vi "CAN Frame Filter.vi"(10 "Filter":T3, 11 "frames in":T4[](array[typedef]) {"payload" format="%x"; "timestamp" format="%<%.7X\n%x>T"; "type" items=["CAN Data"=0, "CAN Remote"=1, "CAN Bus Error"=2, "CAN 2.0 Data"=8, "CAN FD Data"=16, "CAN FD+BRS Data"=24, "J1939 Data"=192, "Delay"=224, "Log Trigger"=225, "Start Trigger"=226]; "identifier" format="%x"}) -> (3 "frames out":T4[](array[typedef]) {"payload" format="%x"; "timestamp" format="%<%.7X\n%x>T"; "type" items=["CAN Data"=0, "CAN Remote"=1, "CAN Bus Error"=2, "CAN 2.0 Data"=8, "CAN FD Data"=16, "CAN FD+BRS Data"=24, "J1939 Data"=192, "Delay"=224, "Log Trigger"=225, "Start Trigger"=226]; "identifier" format="%x"})   [LabVIEW 2019, in "CAN Stream Support Engine.lvlib"]
uses:
  CAN Stream Support Engine.lvlib
  <vilib>/xnet/xnet.llb/XNET Frame CAN.ctl
  <vilib>/xnet/xnet.llb/XNET Frame Type CAN.ctl
  Addon Shared/Types/Direction Filter.ctl
  Addon Shared/Types/Type Filter.ctl
  Addon Shared/CAN Stream Support Shared.lvlib
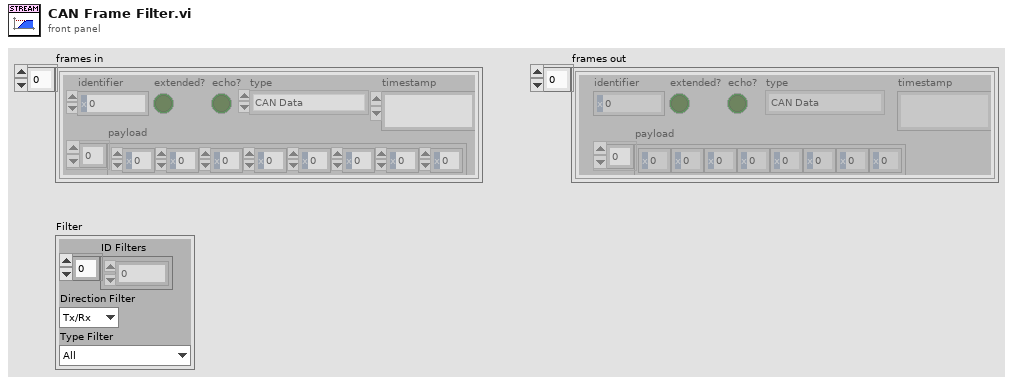
[diagram p1: front panel]
types:
  T1 = typedef "CAN Stream Support Shared.lvlib/Direction Filter.ctl" = enum16{"Tx/Rx", "Rx", "Tx"}
  T2 = typedef "CAN Stream Support Shared.lvlib/Type Filter.ctl" = enum16{"All", "CAN Data", "CAN Remote", "CAN Bus Error", "CAN 2.0 Data", "CAN FD Data", "CAN FD+BRS Data", "J1939 Data", "Delay", "Log Trigger", "Start Trigger"}
  T3 = cluster{"ID Filters":u32[], "Direction Filter":T1, "Type Filter":T2}
  T4 = typedef "XNET Frame CAN.ctl" = cluster{"timestamp":timestamp, "payload":u8[], "identifier":u32, "type":T5, "extended?":bool, "echo?":bool}
  T5 = typedef "XNET Frame Type CAN.ctl" = u8
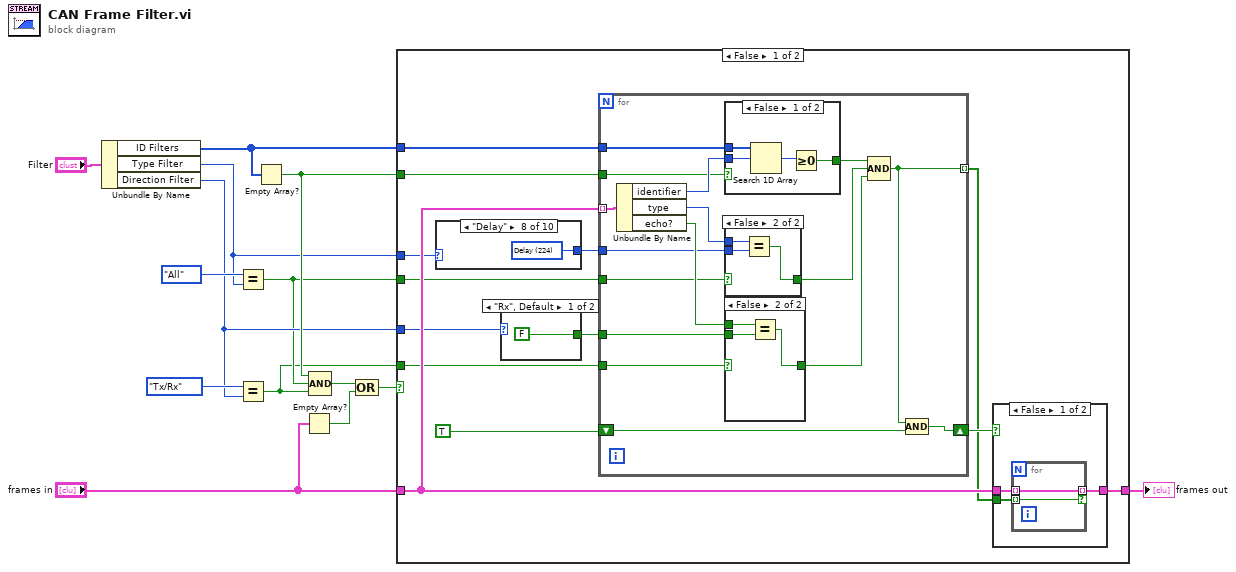
[diagram p0: block diagram]
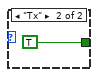
[diagram p2: hidden frame]
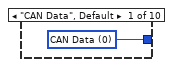
[diagram p3: hidden frame]
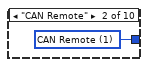
[diagram p4: hidden frame]
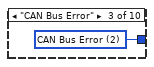
[diagram p5: hidden frame]
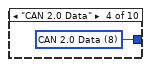
[diagram p6: hidden frame]
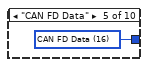
[diagram p7: hidden frame]
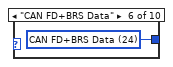
[diagram p8: hidden frame]
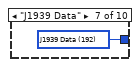
[diagram p9: hidden frame]
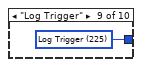
[diagram p10: hidden frame]
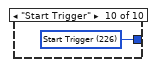
[diagram p11: hidden frame]
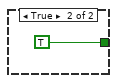
[diagram p13: hidden frame]
diagram:
  n1 = Unbundle By Name("Filter") -> ("ID Filters"=w5:u32[], "Type Filter"=w3:T2, "Direction Filter"=w4:T1)
  n2 = Equal?(x=Type_Filter."All", y=w3) -> (x = y?=w2:bool)
  n3 = Equal?(x=Direction_Filter."Tx/Rx", y=w4) -> (x = y?=w1:bool)
  n4 = Empty Array?(array=w5) -> (empty?=w10:bool)
  n5 = Empty Array?(array="frames in") -> (empty?=w12:bool)
  n6 = Compound Arithmetic op=AND(w10, w2, w1) -> (w13:bool)
  n7 = Compound Arithmetic op=OR(w13, w12) -> (w14:bool)
  n8 = case shown="False" w14 {
    tunnel: [w25 w75] -> w7
    tunnel: "frames in" -> [w24 w75]
    tunnel: w5 -> [w22 _]
    tunnel: w3 -> [w20 _]
    tunnel: w4 -> [w17 _]
    tunnel: w10 -> [w21 _]
    tunnel: w2 -> [w19 _]
    tunnel: w1 -> [w15 _]
    frame False {
      n9 = case shown="\"Delay\"" w20 {
        tunnel: [w30 w31 w32 w33 w34 w35 w36 w37 w38 w39] -> w18
        frame "CAN Data", Default {
          w30 = T5 0 items=["CAN Data"=0, "CAN Remote"=1, "CAN Bus Error"=2, "CAN 2.0 Data"=8, "CAN FD Data"=16, "CAN FD+BRS Data"=24, "J1939 Data"=192, "Delay"=224, "Log Trigger"=225, "Start Trigger"=226] ("Type")
        }
        frame "CAN Remote" {
          w31 = T5 1 items=["CAN Data"=0, "CAN Remote"=1, "CAN Bus Error"=2, "CAN 2.0 Data"=8, "CAN FD Data"=16, "CAN FD+BRS Data"=24, "J1939 Data"=192, "Delay"=224, "Log Trigger"=225, "Start Trigger"=226] ("Type")
        }
        frame "CAN Bus Error" {
          w32 = T5 2 items=["CAN Data"=0, "CAN Remote"=1, "CAN Bus Error"=2, "CAN 2.0 Data"=8, "CAN FD Data"=16, "CAN FD+BRS Data"=24, "J1939 Data"=192, "Delay"=224, "Log Trigger"=225, "Start Trigger"=226] ("Type")
        }
        frame "CAN 2.0 Data" {
          w33 = T5 8 items=["CAN Data"=0, "CAN Remote"=1, "CAN Bus Error"=2, "CAN 2.0 Data"=8, "CAN FD Data"=16, "CAN FD+BRS Data"=24, "J1939 Data"=192, "Delay"=224, "Log Trigger"=225, "Start Trigger"=226] ("Type")
        }
        frame "CAN FD Data" {
          w34 = T5 16 items=["CAN Data"=0, "CAN Remote"=1, "CAN Bus Error"=2, "CAN 2.0 Data"=8, "CAN FD Data"=16, "CAN FD+BRS Data"=24, "J1939 Data"=192, "Delay"=224, "Log Trigger"=225, "Start Trigger"=226] ("Type")
        }
        frame "CAN FD+BRS Data" {
          w35 = T5 24 items=["CAN Data"=0, "CAN Remote"=1, "CAN Bus Error"=2, "CAN 2.0 Data"=8, "CAN FD Data"=16, "CAN FD+BRS Data"=24, "J1939 Data"=192, "Delay"=224, "Log Trigger"=225, "Start Trigger"=226] ("Type")
        }
        frame "J1939 Data" {
          w36 = T5 192 items=["CAN Data"=0, "CAN Remote"=1, "CAN Bus Error"=2, "CAN 2.0 Data"=8, "CAN FD Data"=16, "CAN FD+BRS Data"=24, "J1939 Data"=192, "Delay"=224, "Log Trigger"=225, "Start Trigger"=226] ("Type")
        }
        frame "Delay" {
          w37 = T5 224 items=["CAN Data"=0, "CAN Remote"=1, "CAN Bus Error"=2, "CAN 2.0 Data"=8, "CAN FD Data"=16, "CAN FD+BRS Data"=24, "J1939 Data"=192, "Delay"=224, "Log Trigger"=225, "Start Trigger"=226] ("Type")
        }
        frame "Log Trigger" {
          w38 = T5 225 items=["CAN Data"=0, "CAN Remote"=1, "CAN Bus Error"=2, "CAN 2.0 Data"=8, "CAN FD Data"=16, "CAN FD+BRS Data"=24, "J1939 Data"=192, "Delay"=224, "Log Trigger"=225, "Start Trigger"=226] ("Type")
        }
        frame "Start Trigger" {
          w39 = T5 226 items=["CAN Data"=0, "CAN Remote"=1, "CAN Bus Error"=2, "CAN 2.0 Data"=8, "CAN FD Data"=16, "CAN FD+BRS Data"=24, "J1939 Data"=192, "Delay"=224, "Log Trigger"=225, "Start Trigger"=226] ("Type")
        }
      }
      n10 = case shown="\"Rx\", Default" w17 {
        tunnel: [FALSE ("y") TRUE ("y")] -> w16
        frame "Rx", Default {
        }
        frame "Tx" {
        }
      }
      n11 = for {
        tunnel: w22 -> [w55]
        tunnel: w24 -> [w49] mode=indexing
        tunnel: [w48] -> w23 mode=indexing
        shift-right: [w46] -> w26
        shift-left: TRUE -> [w47]
        tunnel: w19 -> [w44]
        tunnel: w21 -> [w45]
        tunnel: w18 -> [w42]
        tunnel: w16 -> [w41]
        tunnel: w15 -> [w40]
        n12 = Unbundle By Name(w49) -> ("identifier"=w54:u32, "type"=w43:T5, "echo?"=w53:bool)
        n13 = case shown="False" w45 {
          tunnel: w55 -> [w63 _]
          tunnel: w54 -> [w62 _]
          tunnel: [w60 TRUE] -> w50
          frame False {
            n14 = Search 1D Array(1D array=w63, element=w62) -> (index of element=w61:i32)  [unwired: 1 in]
            n15 = Greater Or Equal To 0?(x=w61) -> (x >= 0?=w60:bool)
          }
          frame True {
          }
        }
        n16 = case shown="False" w44 {
          selector: w44 -> [w56 _]
          tunnel: [w56 w59] -> w51
          tunnel: w43 -> [_ w58]
          tunnel: w42 -> [_ w57]
          frame True {
          }
          frame False {
            n17 = Equal?(x=w58, y=w57) -> (x = y?=w59:bool)
          }
        }
        n18 = case shown="False" w40 {
          selector: w40 -> [w65 _]
          tunnel: w53 -> [_ w68]
          tunnel: [w65 w67] -> w52
          tunnel: w41 -> [_ w66]
          frame True {
          }
          frame False {
            n19 = Equal?(x=w68, y=w66) -> (x = y?=w67:bool)
          }
        }
        n20 = Compound Arithmetic op=AND(w50, w51, w52) -> (w48:bool)
        n21 = Compound Arithmetic op=AND(w48, w47) -> (w46:bool)
      }
      n22 = case shown="False" w26 {
        tunnel: w24 -> [w69 w74]
        tunnel: [w70 w74] -> w25
        tunnel: w23 -> [w71 _]
        frame False {
          n23 = for {
            tunnel: w71 -> [w72] mode=indexing
            tunnel: [w73] -> w70 mode=indexing if=w72
            tunnel: w69 -> [w73] mode=indexing
          }
        }
        frame True {
        }
      }
    }
    frame True {
    }
  }
  "frames out" <- w7
